vi "Global Data.vi"() -> ()   [LabVIEW 2024, in "General Type Definitions.lvlib"]
uses:
  General Type Definitions.lvlib
  Device Data.ctl
  Device OS.ctl
panel:
  in  "Device Visualization":i32[](array[numeric])=[0, 2]
  out "Omit RTEXE Results":bool
  out "Omit App SSH Results":bool
  out "Linux TCP":map{string, string}(c390)
  out "Win TCP":map{string, string}(c390)
  out "End of Scan":bool
  out "Timeout":bool
  out "Existing Devices Table":string[][](table)
  in  "Current Device":T1
  # "Data Base"
  # "View Settings"
  # "Session Scanner"
  # "Hardware Selection"
  # "0 -> Hostname\n1 -> Alias\n2 -> IP Address"
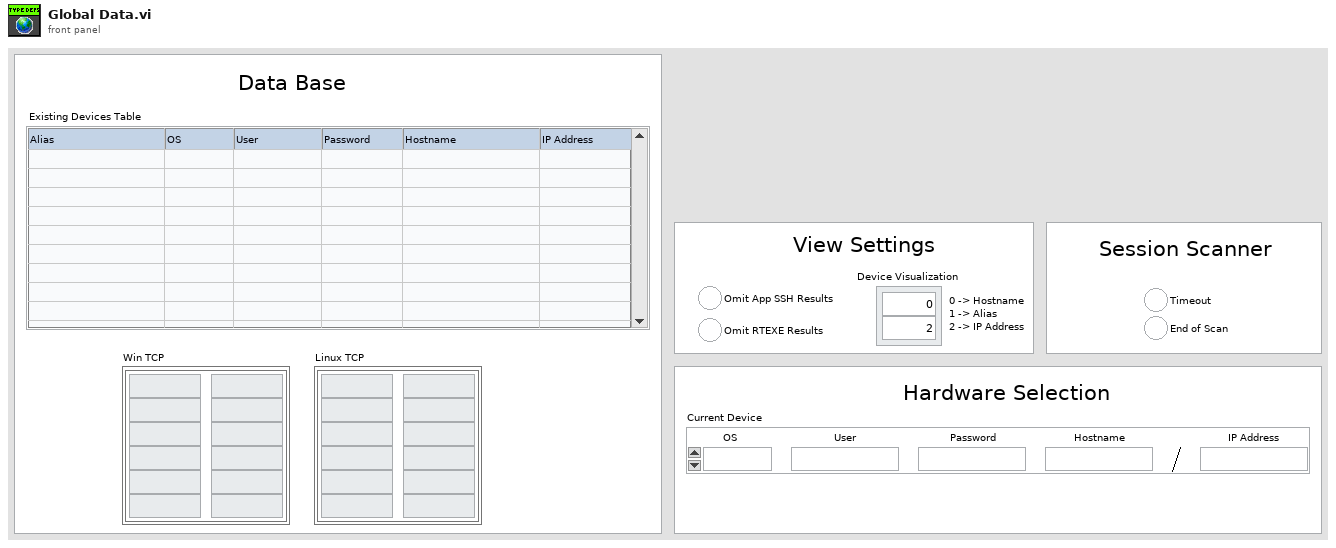
[diagram p1: front panel]
types:
  T1 = typedef "General Type Definitions.lvlib/Device Data.ctl" = cluster{"OS":T2, "User":string, "Password":string, "Hostname":string, "IP Address":string}
  T2 = typedef "General Type Definitions.lvlib/Device OS.ctl" = enum16{"Windows", "Linux"}
diagram:
